vi "SimpleModel.vi"(0 "Links not in joints":T3[](array[typedef]), 2 "Joints":T1[](array[typedef]), 3 "Name":string) -> (4 "urdf out":string)   [LabVIEW 2010]
uses:
  LINK.ctl
  JointTypes.ctl
  JOINT.ctl
panel:
  # "transmission and gazebo"
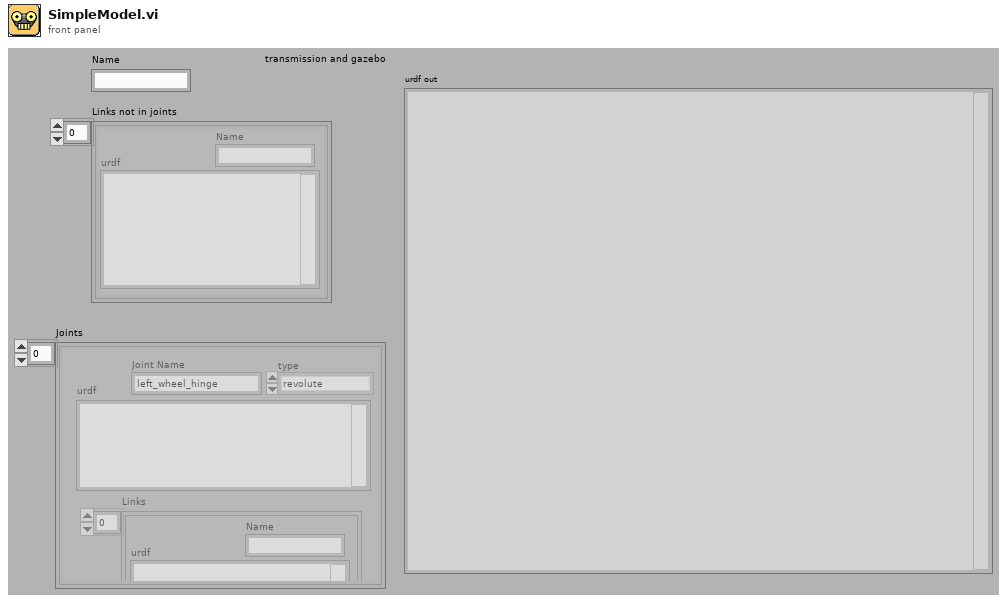
[diagram p1: front panel]
types:
  T1 = typedef "JOINT.ctl" = cluster{"Joint Name":string, "type":T2, "urdf ":string, "Links":T3[]}
  T2 = typedef "JointTypes.ctl" = enum16{"revolute", "continuous", "prismatic", "fixed", "floating", "planar"}
  T3 = typedef "LINK.ctl" = cluster{"Name":string, "urdf":string}
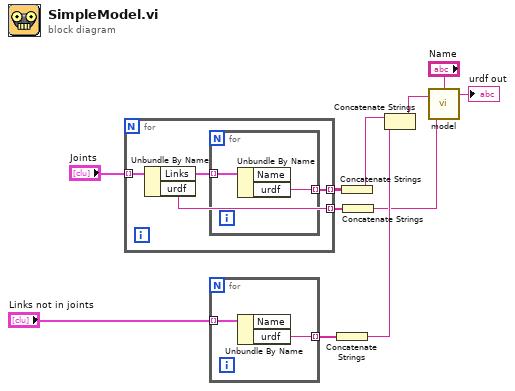
[diagram p0: block diagram]
diagram:
  n1 = for {
    tunnel: "Joints" -> [w15] mode=indexing
    tunnel: [w13] -> w10 mode=indexing
    tunnel: [w12] -> w7 mode=indexing
    n2 = Unbundle By Name(w15) -> ("Links"=w14:T3[], "urdf"=w12:string)
    n3 = for {
      tunnel: w14 -> [w17] mode=indexing
      tunnel: [w16] -> w13 mode=indexing
      n4 = Unbundle By Name(w17) -> ("urdf"=w16:string)  [unwired: 1 out]
    }
  }
  n5 = for {
    tunnel: "Links not in joints" -> [w19] mode=indexing
    tunnel: [w18] -> w8 mode=indexing
    n6 = Unbundle By Name(w19) -> ("urdf"=w18:string)  [unwired: 1 out]
  }
  n7 = Concatenate Strings(w8) -> (w5:string)
  n8 = Concatenate Strings(w10) -> (w6:string)
  n9 = Concatenate Strings(w7) -> (w3:string)
  n10 = Concatenate Strings(w6, w5) -> (w4:string)
  n11 = call "model.vi"("Joints.urdf"=w3, "Links.urdf"=w4, "Name"="Name") -> ("urdf out"=→"urdf out":string)  [unwired: 1 in]
